vi "Handle Command.vi"(8 "error in (no error)":errorcluster, 9 "Data":variant, 10 "Command":string, 11 "Example Instrument in":refnum<class "ExampleInstrument.lvclass">) -> (0 "error out":errorcluster, 1 "Processed Data":variant, 2 "Command":string, 3 "Example Instrument out":refnum<class "ExampleInstrument.lvclass">)   [LabVIEW 2016, in "ExampleInstrument.lvclass"]
uses:
  ExampleInstrument.lvclass
  <userlib>/LevyLab/Levylab Instruments/SMOs/Instrument/Instrument.lvclass
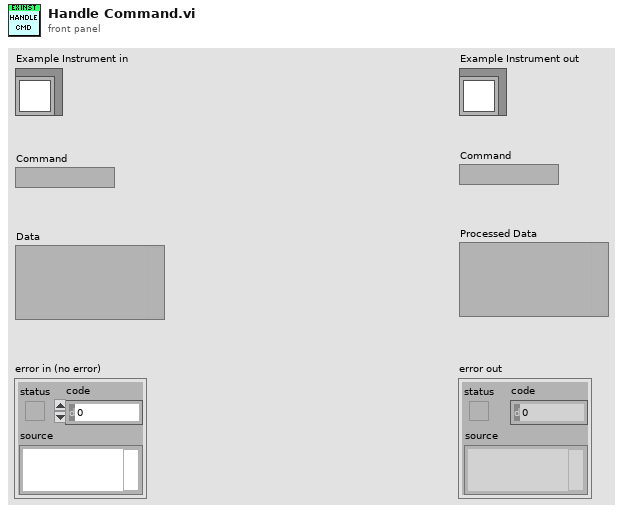
[diagram p1: front panel]
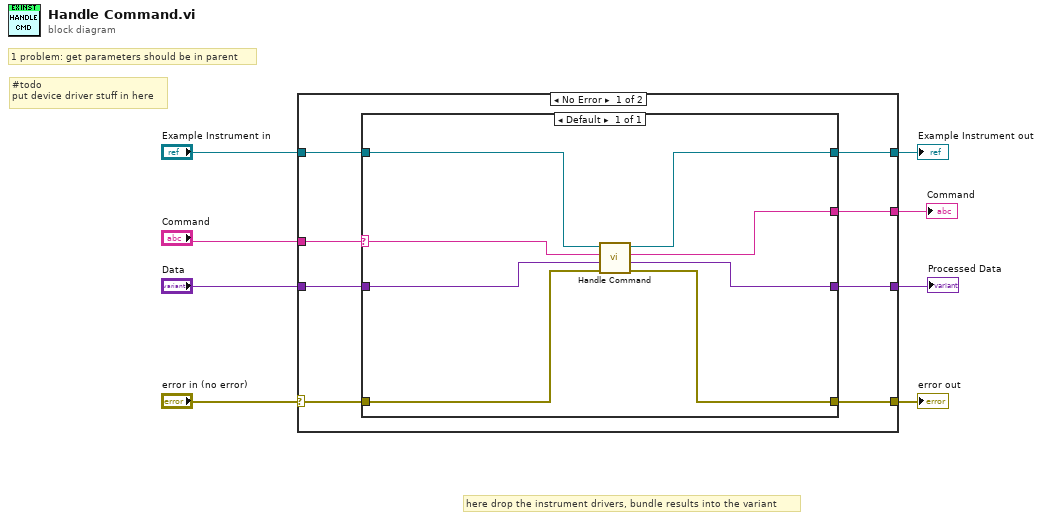
[diagram p0: block diagram]
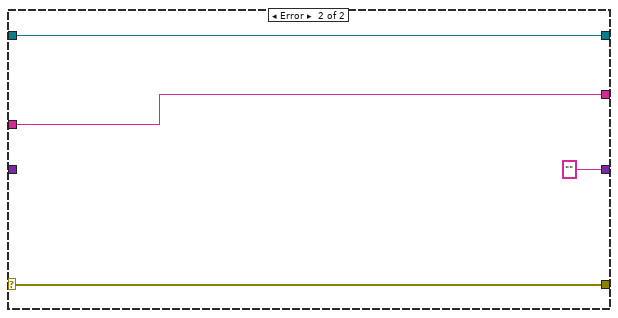
[diagram p2: hidden frame]
diagram:
  # "here drop the instrument drivers, bundle results into the variant"
  # "1 problem: get parameters should be in parent"
  # "#todo\nput device driver stuff in here"
  n1 = case shown="No Error" "error in (no error)" {
    selector: "error in (no error)" -> [w12 w28]
    tunnel: [w10 w28] -> w6
    tunnel: [w14 w27] -> w5
    tunnel: "Example Instrument in" -> [w15 w27]
    tunnel: "Command" -> [w16 w25]
    tunnel: [w13 "" ("String")] -> w3
    tunnel: "Data" -> [w11 _]
    tunnel: [w9 w25] -> w1
    frame No Error {
      n2 = case shown="Default" w16 {
        selector: w16 -> [w24]
        tunnel: w15 -> [w21]
        tunnel: [w18] -> w14
        tunnel: [w20] -> w13
        tunnel: w12 -> [w22]
        tunnel: w11 -> [w23]
        tunnel: [w19] -> w10
        tunnel: [w17] -> w9
        frame Default {
          n3 = call-parent "Handle Command.vi"("error in (no error)"=w22, "Data"=w23, "Command"=w24, "Instrument in"=w21) -> ("error out"=w19:errorcluster, "Processed Data"=w20:variant, "Command"=w17:string, "Instrument out"=w18:refnum<class "ExampleInstrument.lvclass">)  [unwired: 4 in]
        }
      }
    }
    frame Error {
    }
  }
  "error out" <- w6
  "Example Instrument out" <- w5
  "Command" <- w1
  "Processed Data" <- w3
